vi "S7-TCP_READ.vi"(5 "DB Block":u16, 7 "RegisterType":T1=132 items=["I/O (P)"=128, "Input (I)"=129, "Output (Q)"=130, "Bit Memory (M)"=131, "Data (DB)"=132, "Instance Data (DI)"=133, "Local Data (L)"=134, "Predecessor Local Data (VL)"=135], 8 "error in (no error)":errorcluster caption="错误输入（无错误）", 9 "Length":u16, 10 "StartAddress":u32, 11 "S7-TCP 输入":refnum<class "S7-TCP.lvclass">) -> (0 "error out":errorcluster caption="错误输出", 1 "DataValid":bool, 2 "ReadData":u8[](array[numeric]), 3 "S7-TCP 输出":refnum<class "S7-TCP.lvclass">)   [LabVIEW 2018, in "S7-TCP.lvclass"]
uses:
  S7-TCP.lvclass
  Controls/RegisterType.ctl
  S7-TCP.lvclass/S7-TCP.ctl
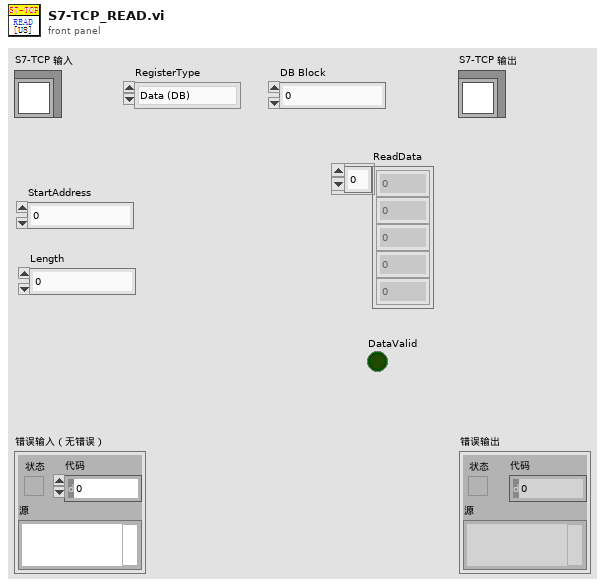
[diagram p1: front panel]
types:
  T1 = typedef "S7-TCP.lvclass/RegisterType.ctl" = u8
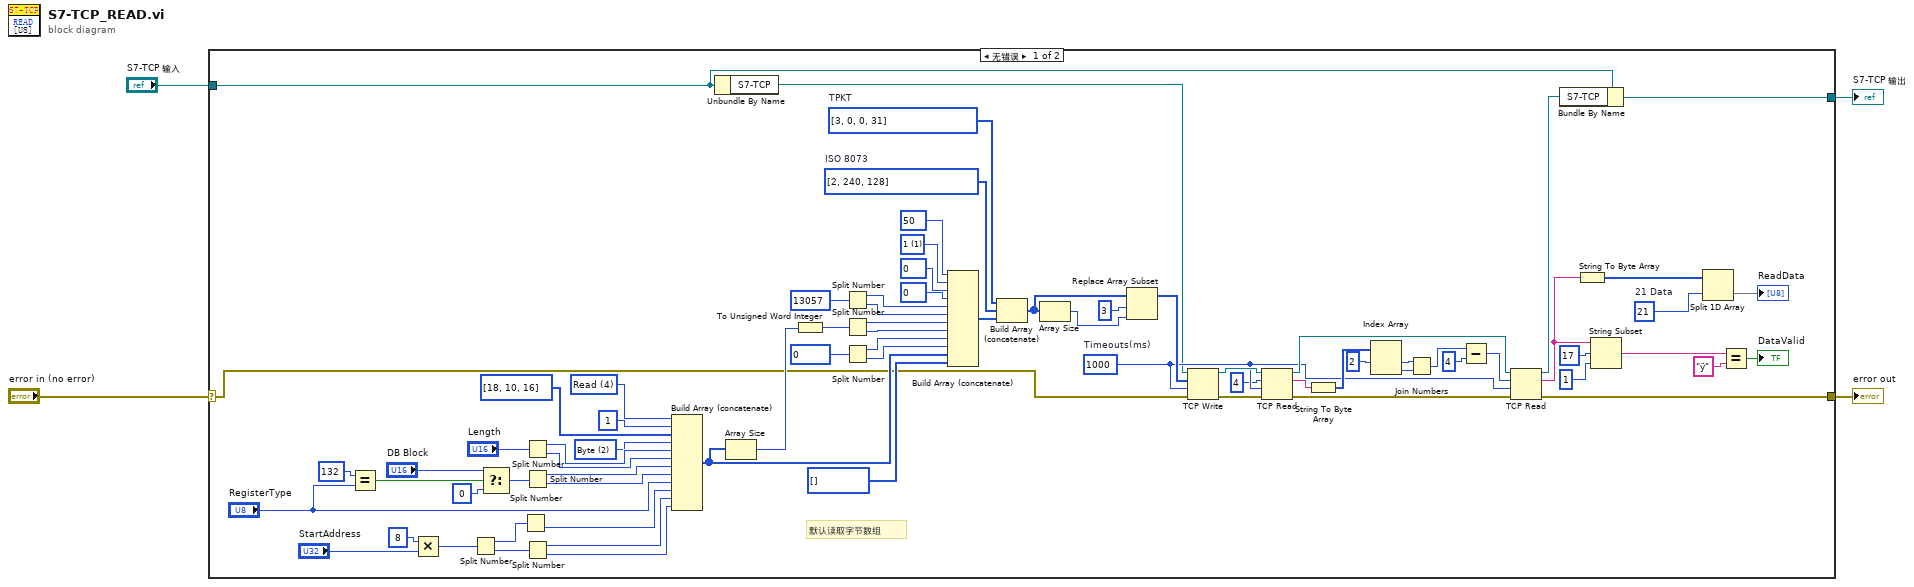
[diagram p0: block diagram]
diagram:
  n1 = case shown="无错误" "error in (no error)" {
    selector: "error in (no error)" -> [w9 w81]
    tunnel: [w5 w81] -> w3
    tunnel: [w7 w80] -> w1
    tunnel: "S7-TCP 输入" -> [w79 w80]
    frame No Error {
      w34 = 21  # 21 Data
      w28 = u32 1000  # Timeouts(ms)
      w27 = u8[] [3, 0, 0, 31]  # TPKT
      w26 = u8[] [2, 240, 128]  # ISO 8073
      w22 = u8 1 items=["1"=1, "2"=2, "3"=3, "7"=7]
      w15 = u8 4 items=["Read"=4, "Write"=5] ("Read / Write")
      w12 = u8 2 items=["Bit"=1, "Byte"=2, "Word"=4, "Dword"=6] ("Transport Type")
      # "默认读取字节数组"
      n2 = Equal?(x=u8 132, y="RegisterType") -> (x = y?=w50:bool)
      n3 = Multiply(x=u32 8 ("y"), y="StartAddress") -> (x*y=w55:u32)
      n4 = Split Number(x=w55) -> (hi(x)=w44:u16, lo(x)=w45:u16)
      n5 = Select(t="DB Block", s=w50, f=u16 0 ("Sequence #")) -> (s? t:f=w53:u16)
      n6 = Split Number(x=w44) -> (lo(x)=w47:u8)  [unwired: 1 out]
      n7 = Split Number(x="Length") -> (hi(x)=w46:u8, lo(x)=w54:u8)
      n8 = Split Number(x=w53) -> (hi(x)=w52:u8, lo(x)=w51:u8)
      n9 = Split Number(x=w45) -> (hi(x)=w48:u8, lo(x)=w49:u8)
      n10 = Build Array (concatenate)(w15, u8 1 ("Sequence #"), u8[] [18, 10, 16] ("Msg Header"), w12, w46, w54, w52, w51, "RegisterType", w47, w48, w49) -> (w42:T1[])
      n11 = Unbundle By Name(w79) -> ("S7-TCP"=w8:refnum<k5>)
      n12 = Array Size(array=w42) -> (size(s)=w62:i32)
      n13 = To Unsigned Word Integer(number=w62) -> (unsigned 16bit integer=w63:u16)
      n14 = Split Number(x=u16 13057 ("DLE")) -> (hi(x)=w60:u8, lo(x)=w61:u8)
      n15 = Split Number(x=w63) -> (hi(x)=w56:u8, lo(x)=w57:u8)
      n16 = Split Number(x=u16 0 ("DLE")) -> (hi(x)=w58:u8, lo(x)=w59:u8)
      n17 = Build Array (concatenate)(u8 50 ("DLE"), w22, u8 0 ("DLE"), u8 0 ("DLE"), w60, w61, w56, w57, w58, w59, w42, u8[] []) -> (w64:T1[])
      n18 = Build Array (concatenate)(w27, w26, w64) -> (w43:T1[])
      n19 = Array Size(array=w43) -> (size(s)=w41:i32)
      n20 = Replace Array Subset(array=w43, new element=w41, index=3) -> (w40:T1[])
      n21 = TCP Write(connection ID=w8, data in=w40, error in (no error)=w9, 9:w28) -> (connection ID out=w38:refnum<k5>, error out=w39:errorcluster)  [unwired: 1 out]
      n22 = TCP Read(connection ID=w38, bytes to read=4, error in (no error)=w39, 9:w28) -> (connection ID out=w71:refnum<k5>, data out=w72:string, error out=w73:errorcluster)  [unwired: 1 in]
      n23 = String To Byte Array(string=w72) -> (unsigned byte array=w66:u8[])
      n24 = Index Array(array=w66, index #1=2 ("索引")) -> (element #1=w67:u8, element #2=w68:u8)  [unwired: 1 in]
      n25 = Join Numbers(hi=w67, lo=w68) -> ((hi.lo)=w69:u16)
      n26 = Subtract(x=w69, y=u16 4) -> (x-y=w70:u16)
      n27 = TCP Read(connection ID=w71, bytes to read=w70, error in (no error)=w73, 9:w28) -> (connection ID out=w6:refnum<k5>, data out=w75:string, error out=w5:errorcluster)  [unwired: 1 in]
      n28 = Bundle By Name(cluster=w79, "S7-TCP"=w6) -> (w7:refnum<class "S7-TCP.lvclass">)
      n29 = String To Byte Array(string=w75) -> (unsigned byte array=w77:u8[])
      n30 = String Subset(string=w75, offset (0)=17 ("偏移量(0)"), length (rest)=1 ("长度（剩余）")) -> (substring=w74:string)
      n31 = Split 1D Array ("拆分一维数组")(array=w77, index=w34) -> (second subarray=→"ReadData":u8[])  [unwired: 1 out]
      n32 = Equal?(x=w74, y="ÿ") -> (x = y?=→"DataValid":bool)
    }
    frame Error {
    }
  }
  "error out" <- w3
  "S7-TCP 输出" <- w1
